vi "Get Output Values.vi"(6 "Last request":bool, 8 "error in (no error)":errorcluster, 10 "Number of points":i32, 11 "Spectrum Recorder in":refnum<class "Spectrum Recorder too.lvclass">) -> (0 "error out":errorcluster, 2 "Output values":dbl[](array[numeric]), 3 "Spectrum Recorder out":refnum<class "Spectrum Recorder too.lvclass">)   [LabVIEW 2016, in "Spectrum Recorder too.lvclass"]
uses:
  Spectrum Recorder too.lvclass
  C:/github/Measure_core/Instrument Actor/Instrument Actor.lvclass
  Spectrum Recorder too.lvclass/Spectrum Recorder too.ctl
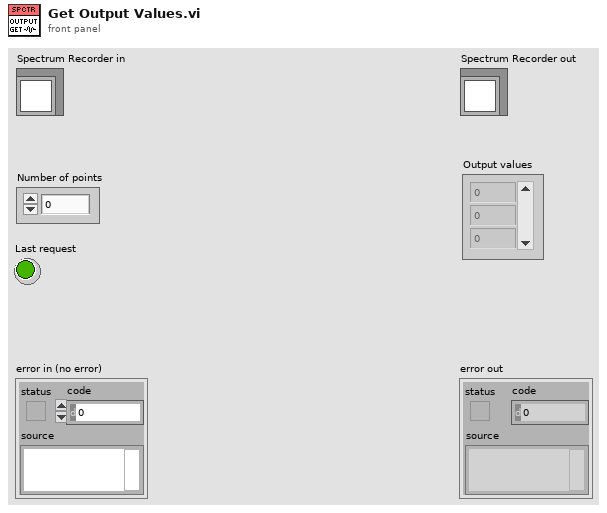
[diagram p1: front panel]
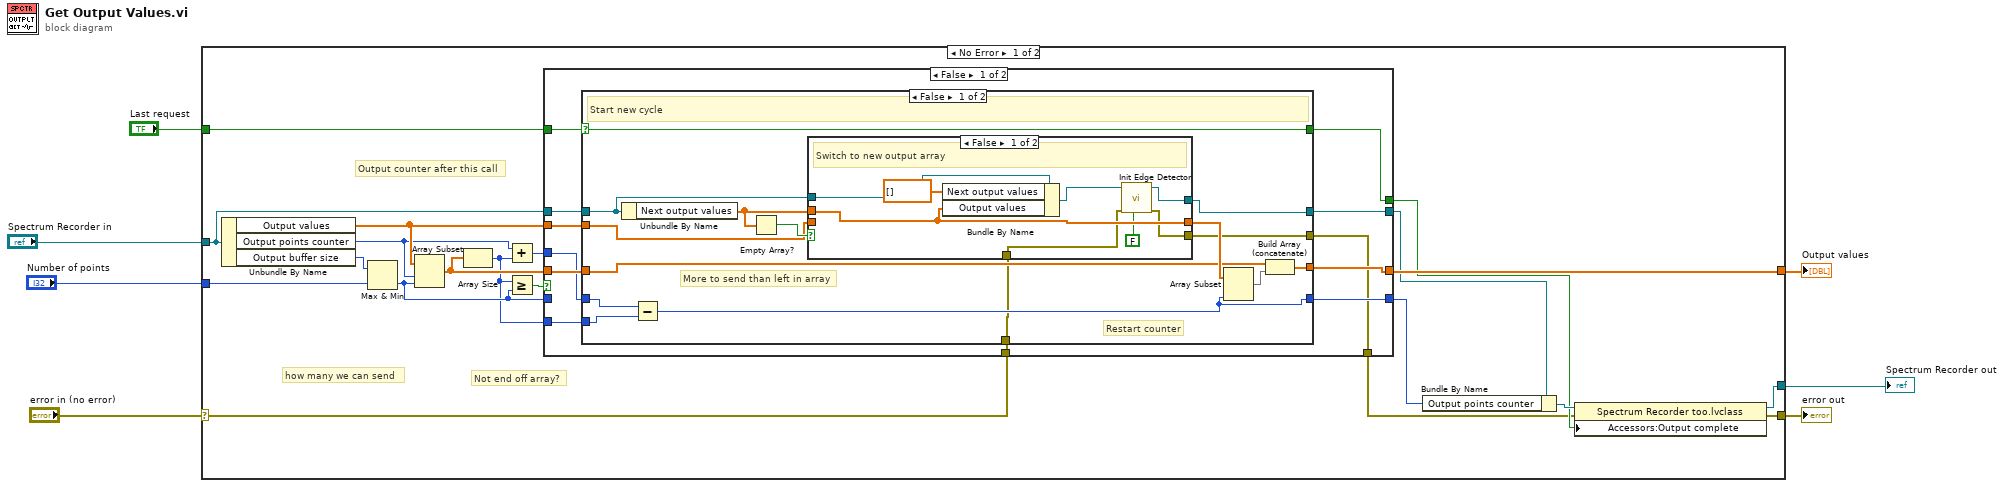
[diagram p0: block diagram]
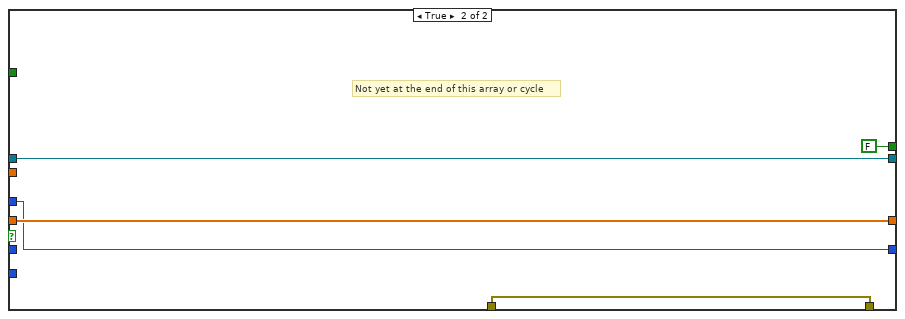
[diagram p4: hidden frame]
diagram:
  n1 = case shown="No Error" "error in (no error)" {
    selector: "error in (no error)" -> [w8 w77]
    tunnel: [w27 w77] -> w6
    tunnel: [w25 w76] -> w4
    tunnel: "Spectrum Recorder in" -> [w22 w76]
    tunnel: "Number of points" -> [w13 _]
    tunnel: [w19 _] -> w2
    tunnel: "Last request" -> [w23 _]
    frame No Error {
      # "Not end off array?"
      # "Output counter after this call"
      # "how many we can send"
      n2 = Unbundle By Name(w22) -> ("Output values"=w20:dbl[], "Output points counter"=w12:i32, "Output buffer size"=w11:i32)
      n3 = Max & Min(x=w11, y=w13) -> (min(x,y)=w21:i32)  [unwired: 1 out]
      n4 = Array Subset(array=w20, index=w12, length=w21) -> (w16:dbl[])
      n5 = Array Size(array=w16) -> (size(s)=w10:i32)
      n6 = Add(x=w12, y=w10) -> (x+y=w15:i32)
      n7 = Greater Or Equal?(x=w10, y=w21) -> (x >= y?=w24:bool)
      n8 = case shown="False" w24 {
        tunnel: w20 -> [w37 _]
        tunnel: w15 -> [w30 w73]
        tunnel: w21 -> [_ _]
        tunnel: w23 -> [w39 _]
        tunnel: w22 -> [w38 w72]
        tunnel: [w35 w74] -> w19
        tunnel: w16 -> [w36 w74]
        tunnel: [w34 FALSE] -> w18
        tunnel: [w33 w73] -> w17
        tunnel: [w32 w72] -> w14
        tunnel: w10 -> [w31 _]
        tunnel: [w29 w71] -> w9
        tunnel: w8 -> [w28 w71]
        frame False {
          n9 = case shown="False" w39 {
            selector: w39 -> [w45 w70]
            tunnel: w38 -> [w53 w68]
            tunnel: w37 -> [w51 _]
            tunnel: w36 -> [w48 w67]
            tunnel: w30 -> [w49 w69]
            tunnel: [w46 w67] -> w35
            tunnel: [w45 w70] -> w34
            tunnel: [w44 w69] -> w33
            tunnel: [w42 w68] -> w32
            tunnel: w31 -> [w43 _]
            tunnel: [w41 w66] -> w29
            tunnel: w28 -> [w40 w66]
            frame False {
              # "Restart counter"
              # "More to send than left in array"
              # "Start new cycle"
              n10 = Unbundle By Name(w53) -> ("Next output values"=w52:dbl[])
              n11 = Subtract(x=w49, y=w43) -> (x-y=w44:i32)
              n12 = Empty Array?(array=w52) -> (empty?=w54:bool)
              n13 = case shown="False" w54 {
                tunnel: w53 -> [w62 w65]
                tunnel: w52 -> [w61 _]
                tunnel: [w58 w65] -> w42
                tunnel: [w61 w64] -> w50
                tunnel: w51 -> [_ w64]
                tunnel: [w57 w63] -> w41
                tunnel: w40 -> [w56 w63]
                frame False {
                  # "Switch to new output array"
                  n14 = Bundle By Name(cluster=w62, "Next output values"=dbl[] [], "Output values"=w61) -> (w59:refnum<class "Spectrum Recorder too.lvclass">)
                  n15 = call-dynamic "Init Edge Detector.vi"("Unsee last word"=FALSE, "error in (no error)"=w56, "Spectrum Recorder too in"=w59) -> ("error out"=w57:errorcluster, "Spectrum Recorder too out"=w58:refnum<class "Spectrum Recorder too.lvclass">)  [unwired: 7 in]
                }
                frame True {
                  # "Repeat same output array"
                }
              }
              n16 = Array Subset(array=w50, length=w44) -> (w47:dbl[])  [unwired: 1 in]
              n17 = Build Array (concatenate)(w48, w47) -> (w46:dbl[])
            }
            frame True {
              # "All output done"
            }
          }
        }
        frame True {
          # "Not yet at the end of this array or cycle"
        }
      }
      n18 = Bundle By Name(cluster=w14, "Output points counter"=w17) -> (w26:refnum<class "Spectrum Recorder too.lvclass">)
      n19 = property class="Spectrum Recorder too.lvclass"(reference=w26, error in=w9, "Accessors:Output complete"=w18) -> (reference out=w25:refnum<class "Spectrum Recorder too.lvclass">, error out=w27:errorcluster)
    }
    frame Error {
    }
  }
  "error out" <- w6
  "Spectrum Recorder out" <- w4
  "Output values" <- w2
